vi "Write ColunmsList.vi"(8 "error in (no error)":errorcluster, 10 "ColunmsList":string[](array[string]), 11 "DataBase_SQL in":refnum<class "DataBase_SQL.lvclass">) -> (0 "error out":errorcluster, 3 "DataBase_SQL out":refnum<class "DataBase_SQL.lvclass">)   [LabVIEW 2021, in "DataBase_SQL.lvclass"]
uses:
  <userlib>/John_Lib/DataBase/DataBase_SQL/DataBase_SQL.lvclass
  <userlib>/John_Lib/DataBase/DataBase_SQL/DataBase_SQL.lvclass/DataBase_SQL.ctl
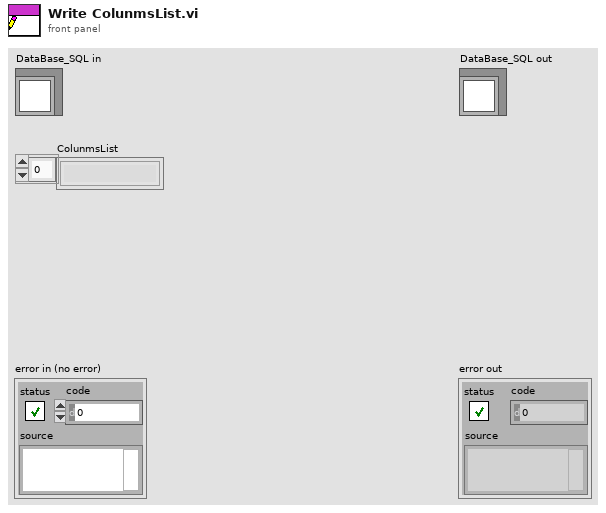
[diagram p1: front panel]
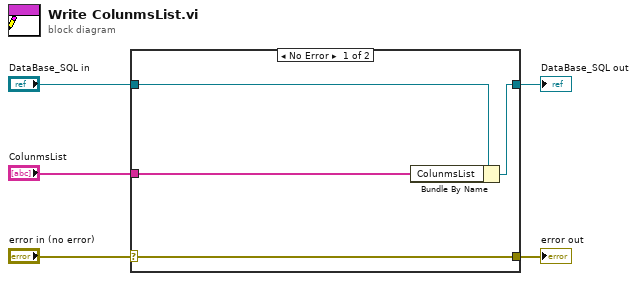
[diagram p0: block diagram]
diagram:
  n1 = case shown="No Error" "error in (no error)" {
    selector: "error in (no error)" -> [w9 w10]
    tunnel: [w9 w10] -> w4
    tunnel: [w7 w11] -> w2
    tunnel: "DataBase_SQL in" -> [w8 w11]
    tunnel: "ColunmsList" -> [w6 _]
    frame No Error {
      n2 = Bundle By Name(cluster=w8, "ColunmsList"=w6) -> (w7:refnum<class "DataBase_SQL.lvclass">)
    }
    frame Error {
    }
  }
  "error out" <- w4
  "DataBase_SQL out" <- w2
